vi "location_plot.vi"() -> ()   [LabVIEW 2016]
uses:
  <vilib>/sound2/lvsound2.llb/Sound Output Task ID.ctl
panel:
  in  "task ID 4":T1 format="%.0x"
  out "task ID out":T1 format="%.0x"
  out "error out 4":errorcluster
  in  "error in (no error) 4":errorcluster
  out "output 12":dbl
  in  "timeout (sec) 3":dbl
  in  "error in (no error) 3":errorcluster
  out "error out 3":errorcluster
  out "task ID 3":T1 format="%.0x"
  in  "timeout (sec) 2":dbl
  in  "error in (no error) 2":errorcluster
  out "error out 2":errorcluster
  out "task ID 2":T1 format="%.0x"
  out "Ball 5":cluster{"Color":string, "y":dbl, "x":dbl}
  out "Ball 4":cluster{"Color":string, "y":dbl, "x":dbl}
  out "Ball 3":cluster{"Color":string, "x":dbl, "y":dbl}
  out "Ball 2":cluster{"Color":string, "x":dbl, "y":dbl}
  out "ballcnt":dbl
  out "Ball 1":cluster{"Color":string, "x":dbl, "y":dbl}
  out "by":dbl
  out "task ID":T1 format="%.0x"
  out "error out":errorcluster
  in  "error in (no error)":errorcluster
  in  "timeout (sec)":dbl
  out "bx":dbl
  out "Numeric 2":dbl
  out "Numeric":dbl
  out "bflag":dbl
  out "pathy":dbl
  out "pathx":dbl
  out "object":dbl
  in  "stop":bool
  in  "Display History":bool
  out "2D Picture":picture
  in  "Size":i16=3
  out "bearing":dbl
  out "velocity":dbl
  out "Y":dbl
  out "X":dbl=5.0
  in  "DAC 2":dbl
  in  "DAC 1":dbl
  in  "Send Button":bool
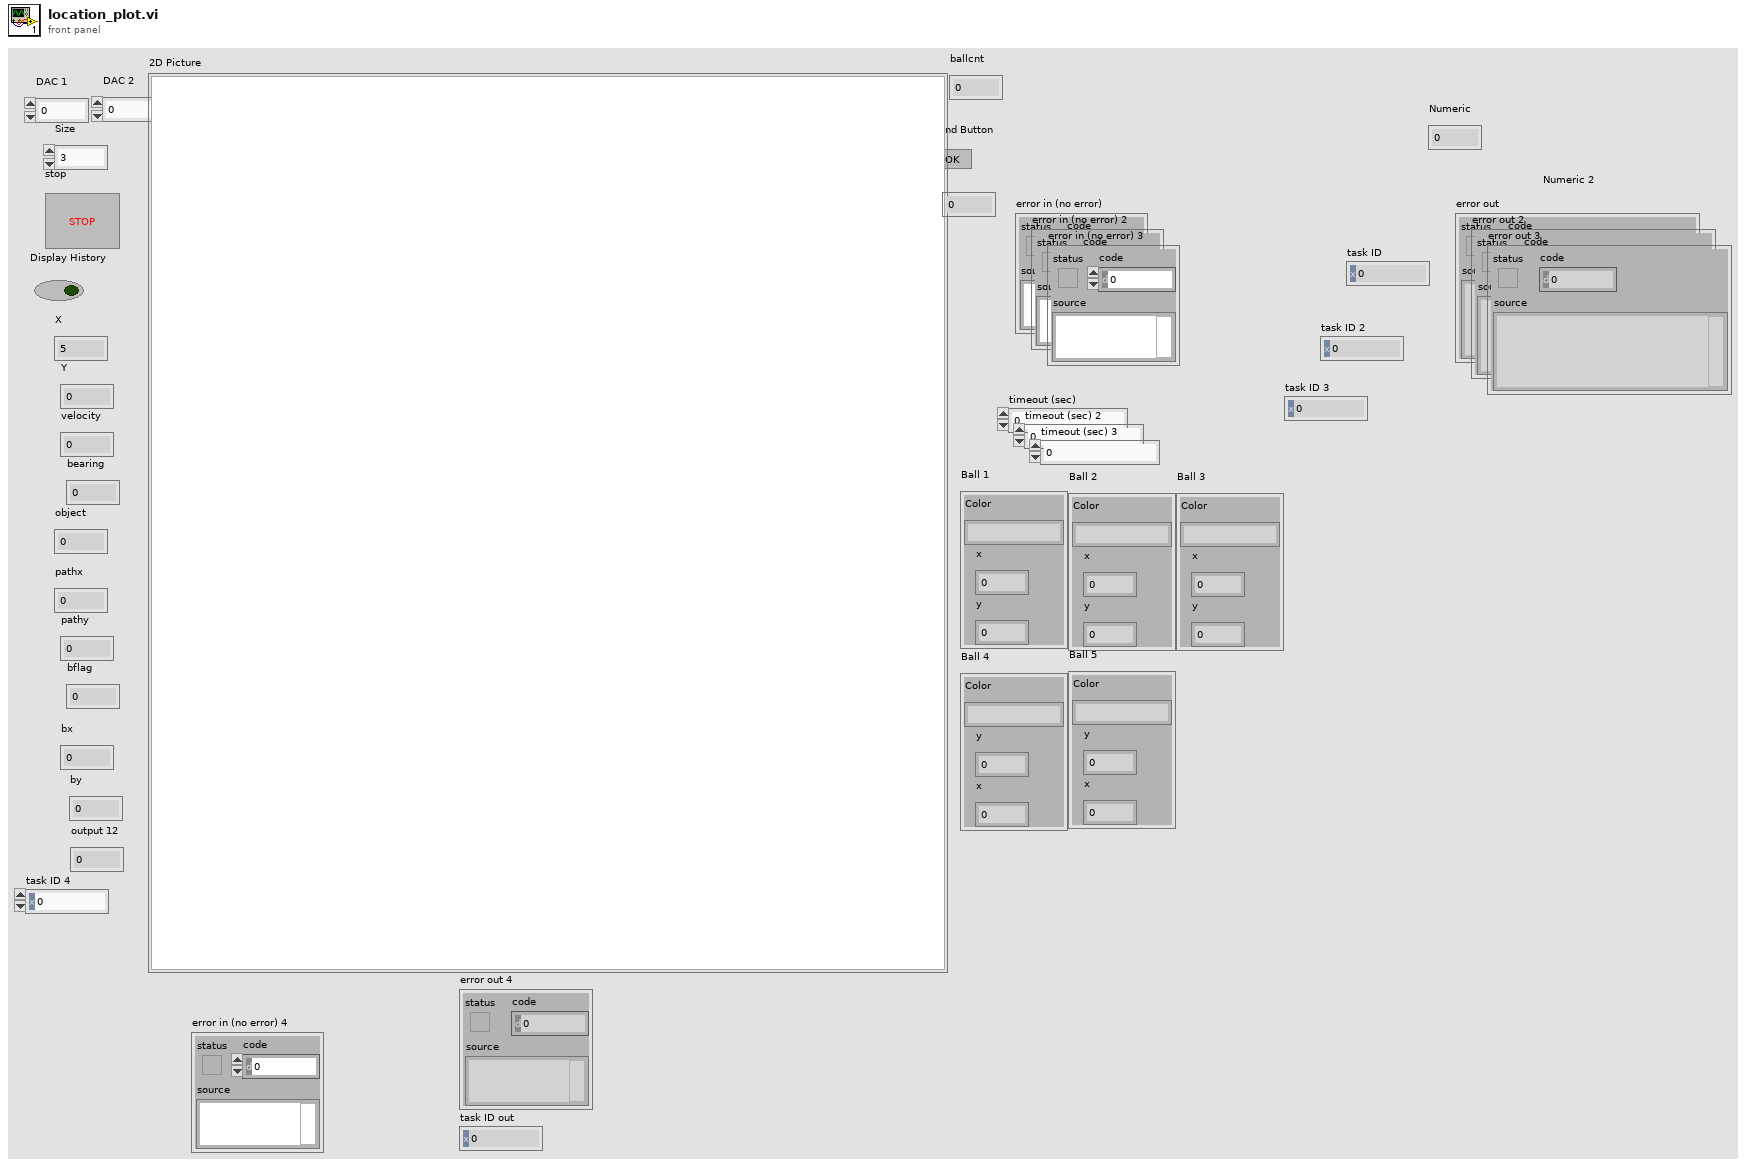
[diagram p1: front panel]
types:
  T1 = typedef "Sound Output Task ID.ctl" = u32
  T2 = cluster{"Width":u16, "Style":enum32{"Solid", "Dash", "Dot", "DashDot", "DashDotDot"}}
  T3 = enum16{"Standard", "Buffered", "CRLF", "Immediate"}
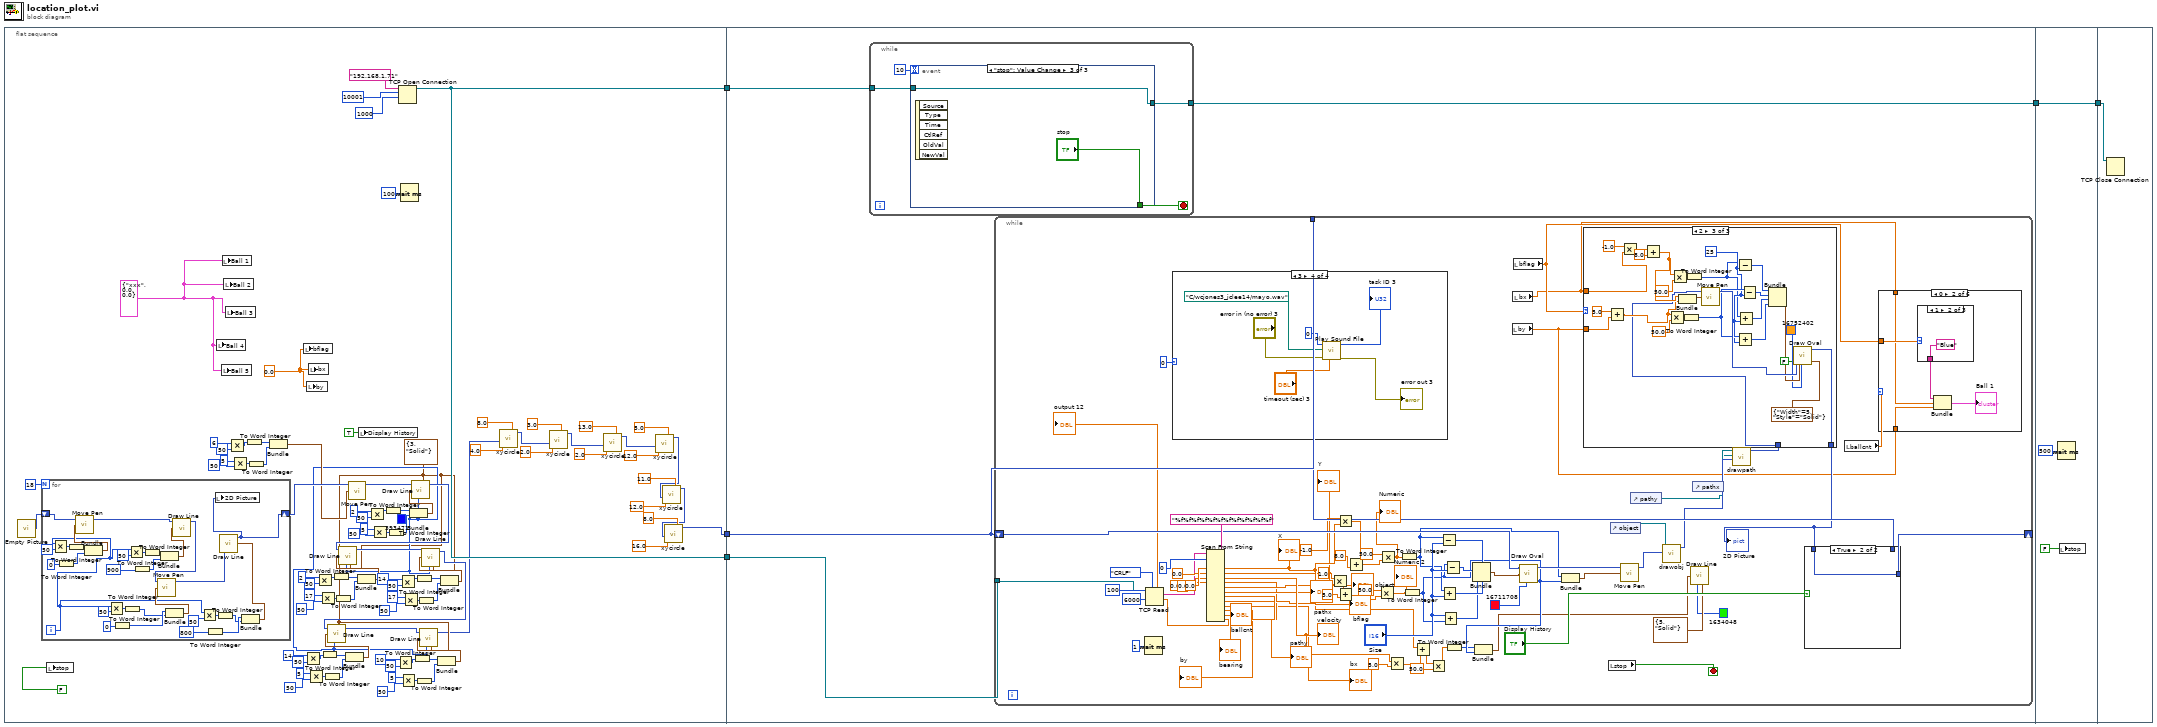
[diagram p0: block diagram]
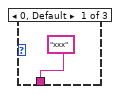
[diagram p3: hidden frame]
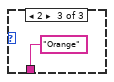
[diagram p4: hidden frame]
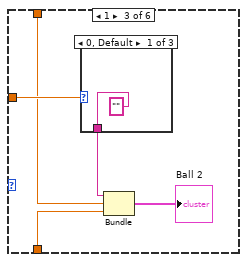
[diagram p5: hidden frame]
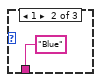
[diagram p6: hidden frame]
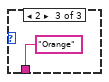
[diagram p7: hidden frame]
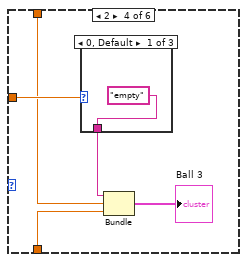
[diagram p8: hidden frame]
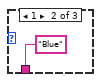
[diagram p9: hidden frame]
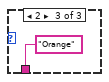
[diagram p10: hidden frame]
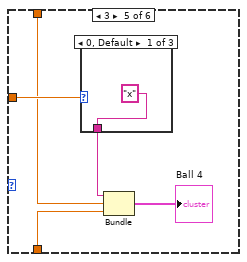
[diagram p11: hidden frame]
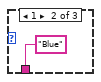
[diagram p12: hidden frame]
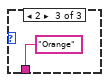
[diagram p13: hidden frame]
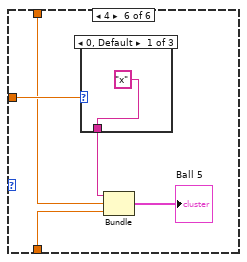
[diagram p14: hidden frame]
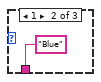
[diagram p15: hidden frame]
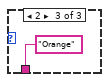
[diagram p16: hidden frame]
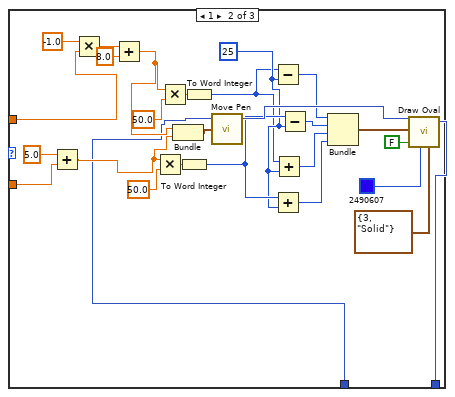
[diagram p18: hidden frame]
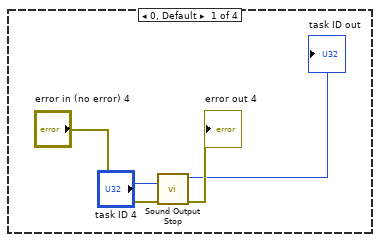
[diagram p19: hidden frame]
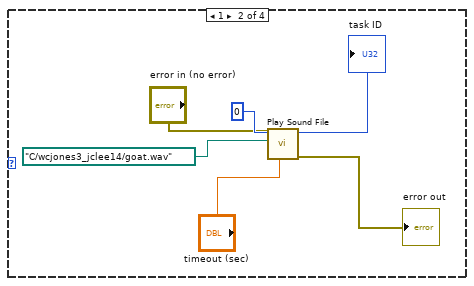
[diagram p20: hidden frame]
diagram:
  n1 = flat-sequence {
    tunnel: [w93] -> w5
    tunnel: [w93] -> w4
    tunnel: [w8] -> w1
    tunnel: w5 -> [w131]
    tunnel: w4 -> [w130]
    tunnel: [w129] -> w3
    tunnel: w1 -> [w128]
    tunnel: w3 -> [w344]
    tunnel: [w344] -> w2
    tunnel: w2 -> [w346]
    frame #0 {
      w6 = cluster{"Color":string, "x":dbl, "y":dbl} {"Color"="xxx", "x"=0.0, "y"=0.0} ("Ball 1")
      w7 = 0.0
      w27 = T2 {"Width"=3, "Style"=enum."Solid"} ("pen")
      w28 = u32 393471 ("color(black)")
      n2 = call "Empty Picture"() -> ("empty picture"=w89:picture)
      n3 = for {
        N: 18 -> [_]
        shift-right: [w100] -> w88
        shift-left: w89 -> [w99]
        i -> [w98]
        n4 = Multiply(x=w98, y=50) -> (x*y=w126:i32)
        n5 = To Word Integer(number=0) -> (16bit integer=w124:i16)
        n6 = To Word Integer(number=w126) -> (16bit integer=w123:i16)
        n7 = Bundle(w123, w124) -> (w122:cluster{i16, i16})  [unwired: 1 in]
        n8 = call <vilib>:"Move Pen.vi"("new position"=w122, "picture"=w99) -> ("new picture"=w115:picture)  [unwired: 3 in]
        n9 = Multiply(x=w98, y=50) -> (x*y=w108:i32)
        n10 = To Word Integer(number=0) -> (16bit integer=w106:i16)
        n11 = To Word Integer(number=w108) -> (16bit integer=w105:i16)
        n12 = Multiply(x=w98, y=50) -> (x*y=w118:i32)
        n13 = To Word Integer(number=900) -> (16bit integer=w120:i16)
        n14 = To Word Integer(number=w118) -> (16bit integer=w121:i16)
        n15 = Bundle(w121, w120) -> (w116:cluster{i16, i16})  [unwired: 1 in]
        n16 = Bundle(w106, w105) -> (w110:cluster{i16, i16})  [unwired: 1 in]
        n17 = call <vilib>:"Draw Line.vi"("picture"=w115, "end point"=w116) -> ("new picture"=w102:picture)  [unwired: 7 in]
        n18 = call <vilib>:"Move Pen.vi"("new position"=w110, "picture"=w102) -> ("new picture"=w101:picture)  [unwired: 3 in]
        n19 = Multiply(x=w98, y=50) -> (x*y=w112:i32)
        n20 = To Word Integer(number=800) -> (16bit integer=w104:i16)
        n21 = To Word Integer(number=w112) -> (16bit integer=w103:i16)
        n22 = Bundle(w104, w103) -> (w114:cluster{i16, i16})  [unwired: 1 in]
        n23 = call <vilib>:"Draw Line.vi"("picture"=w101, "end point"=w114) -> ("new picture"=w100:picture)  [unwired: 7 in]
        n24 = local write "2D Picture"(w100) -> ()
      }
      n25 = local write "stop"(FALSE ("stop")) -> ()
      n26 = local write "Ball 4"(w6) -> ()
      n27 = local write "Ball 5"(w6) -> ()
      n28 = local write "Ball 1"(w6) -> ()
      n29 = local write "Ball 2"(w6) -> ()
      n30 = local write "Ball 3"(w6) -> ()
      n31 = Multiply(x=6, y=50) -> (x*y=w80:i32)
      n32 = Multiply(x=5, y=50) -> (x*y=w85:i32)
      n33 = To Word Integer(number=w80) -> (16bit integer=w86:i16)
      n34 = To Word Integer(number=w85) -> (16bit integer=w87:i16)
      n35 = Bundle(w86, w87) -> (w79:cluster{i16, i16})  [unwired: 1 in]
      n36 = local write "bflag"(w7) -> ()
      n37 = Multiply(x=14, y=50) -> (x*y=w45:i32)
      n38 = local write "by"(w7) -> ()
      n39 = Multiply(x=5, y=50) -> (x*y=w49:i32)
      n40 = local write "bx"(w7) -> ()
      n41 = Multiply(x=2, y=50) -> (x*y=w63:i32)
      n42 = Multiply(x=17, y=50) -> (x*y=w67:i32)
      n43 = To Word Integer(number=w45) -> (16bit integer=w44:i16)
      n44 = To Word Integer(number=w49) -> (16bit integer=w50:i16)
      n45 = To Word Integer(number=w63) -> (16bit integer=w62:i16)
      n46 = To Word Integer(number=w67) -> (16bit integer=w68:i16)
      n47 = Bundle(w44, w50) -> (w43:cluster{i16, i16})  [unwired: 1 in]
      n48 = call <vilib>:"Move Pen.vi"("new position"=w79, "picture"=w88) -> ("new picture"=w78:picture)  [unwired: 3 in]
      n49 = Bundle(w62, w68) -> (w61:cluster{i16, i16})  [unwired: 1 in]
      n50 = local write "Display History"(TRUE ("Display History")) -> ()
      n51 = Multiply(x=2, y=50) -> (x*y=w77:i32)
      n52 = Multiply(x=5, y=50) -> (x*y=w72:i32)
      n53 = To Word Integer(number=w77) -> (16bit integer=w71:i16)
      n54 = To Word Integer(number=w72) -> (16bit integer=w70:i16)
      n55 = Multiply(x=10, y=50) -> (x*y=w35:i32)
      n56 = TCP Open Connection(address="192.168.1.71", remote port or service name=u16 10001, timeout ms (60000)=1000) -> (connection ID=w93:refnum<k5>)  [unwired: 2 in, 1 out]
      n57 = Multiply(x=14, y=50) -> (x*y=w57:i32)
      n58 = Multiply(x=5, y=50) -> (x*y=w31:i32)
      n59 = Wait (ms)(milliseconds to wait=u32 100) -> ()  [unwired: 1 out]
      n60 = Multiply(x=17, y=50) -> (x*y=w53:i32)
      n61 = Bundle(w71, w70) -> (w69:cluster{i16, i16})  [unwired: 1 in]
      n62 = call <vilib>:"Draw Line.vi"("picture"=w78, "end point"=w69, "color(black)"=w28, "pen"=w27) -> ("new picture"=w60:picture)  [unwired: 5 in]
      n63 = call <vilib>:"Draw Line.vi"("picture"=w60, "end point"=w61, "color(black)"=w28, "pen"=w27) -> ("new picture"=w51:picture)  [unwired: 5 in]
      n64 = To Word Integer(number=w35) -> (16bit integer=w36:i16)
      n65 = To Word Integer(number=w57) -> (16bit integer=w58:i16)
      n66 = To Word Integer(number=w31) -> (16bit integer=w30:i16)
      n67 = To Word Integer(number=w53) -> (16bit integer=w52:i16)
      n68 = Bundle(w36, w30) -> (w37:cluster{i16, i16})  [unwired: 1 in]
      n69 = Bundle(w58, w52) -> (w59:cluster{i16, i16})  [unwired: 1 in]
      n70 = call <vilib>:"Draw Line.vi"("picture"=w51, "end point"=w59, "color(black)"=w28, "pen"=w27) -> ("new picture"=w42:picture)  [unwired: 5 in]
      n71 = call <vilib>:"Draw Line.vi"("picture"=w42, "end point"=w43, "color(black)"=w28, "pen"=w27) -> ("new picture"=w29:picture)  [unwired: 5 in]
      n72 = call <vilib>:"Draw Line.vi"("picture"=w29, "end point"=w37, "color(black)"=w28, "pen"=w27) -> ("new picture"=w16:picture)  [unwired: 5 in]
      n73 = call "xycircle.vi"("new picture in"=w16, "y"=4.0, "x"=8.0) -> ("new picture out"=w15:picture)  [unwired: 8 in]
      n74 = call "xycircle.vi"("new picture in"=w15, "y"=2.0, "x"=3.0) -> ("new picture out"=w14:picture)  [unwired: 8 in]
      n75 = call "xycircle.vi"("new picture in"=w14, "y"=2.0, "x"=13.0) -> ("new picture out"=w13:picture)  [unwired: 8 in]
      n76 = call "xycircle.vi"("new picture in"=w13, "y"=12.0, "x"=5.0) -> ("new picture out"=w12:picture)  [unwired: 8 in]
      n77 = call "xycircle.vi"("new picture in"=w12, "y"=12.0, "x"=11.0) -> ("new picture out"=w9:picture)  [unwired: 8 in]
      n78 = call "xycircle.vi"("new picture in"=w9, "y"=16.0, "x"=8.0) -> ("new picture out"=w8:picture)  [unwired: 8 in]
    }
    frame #1 {
      n79 = while {
        tunnel: w131 -> [w326]
        tunnel: [w324] -> w129
        stop <- w327 stop-if-true
        n80 = event shown="[2] \"stop\": Value Change" {
          selector: _ -> [_ _ _]
          dyn-events: _ -> [_ _ _]
          timeout: 10 -> [_ _ _]
          tunnel: [FALSE FALSE "stop"] -> w327
          tunnel: w326 -> [w328 w332 w341]
          tunnel: [w328 w331 w341] -> w324
          event Timeout {
            n81 = event-data() -> ()  [unwired: 1 in, 3 out]
          }
          event "Send Button": Value Change {
            n82 = event-data() -> ()  [unwired: 1 in, 6 out]
            n83 = Format Into String(format string="%f %f", "DAC 1", "DAC 2") -> (resulting string=w337:string)  [unwired: 2 in, 1 out]
            n84 = Concatenate Strings("\\FD" ("string"), w337, "\\FF" ("string")) -> (w334:string)
            n85 = TCP Write(connection ID=w332, data in=w334, 9:100 ("timeout ms (25000)")) -> (connection ID out=w331:refnum<k5>)  [unwired: 1 in, 2 out]
          }
          event "stop": Value Change {
            n86 = event-data() -> ()  [unwired: 1 in, 6 out]
          }
        }
      }
      n87 = while {
        tunnel: w130 -> [w201]
        shift-right: [w183] -> _
        shift-left: w128 -> [w181]
        tunnel: w128 -> [w182]
        stop <- w184 stop-if-true
        n88 = Wait (ms)(milliseconds to wait=u32 1) -> ()  [unwired: 1 out]
        n89 = TCP Read(connection ID=w201, bytes to read=100, 7:T3."CRLF" ("mode (standard)"), 9:6000 ("timeout ms (25000)")) -> (data out=w193:string)  [unwired: 1 in, 2 out]
        n90 = case shown="3" 0 {
          frame 0, Default {
            n91 = call <vilib>:"Sound Output Stop.vi"("error in (no error)"="error in (no error) 4", "task ID"="task ID 4") -> ("error out"=→"error out 4":errorcluster, "task ID out"=→"task ID out":T1)  [unwired: 8 in]
          }
          frame 1 {
            n92 = call <vilib>:"Play Sound File.vi"("timeout (sec)"="timeout (sec)", "error in (no error)"="error in (no error)", "path"=path "C:/wcjones3_jclee14/goat.wav", "device ID"=u32 0) -> ("error out"=→"error out":errorcluster, "task ID"=→"task ID":T1)  [unwired: 6 in]
          }
          frame 2 {
            n93 = call <vilib>:"Play Sound File.vi"("timeout (sec)"="timeout (sec) 2", "error in (no error)"="error in (no error) 2", "path"=path "C:/wcjones3_jclee14/sendit.wav", "device ID"=u32 0) -> ("error out"=→"error out 2":errorcluster, "task ID"=→"task ID 2":T1)  [unwired: 6 in]
          }
          frame 3 {
            n94 = call <vilib>:"Play Sound File.vi"("timeout (sec)"="timeout (sec) 3", "error in (no error)"="error in (no error) 3", "path"=path "C:/wcjones3_jclee14/mayo.wav", "device ID"=u32 0) -> ("error out"=→"error out 3":errorcluster, "task ID"=→"task ID 3":T1)  [unwired: 6 in]
          }
        }
        n95 = Scan From String(format string="%f%f%f%f%f%f%f%f%f%f%f%f", input string=w193, initial scan location=u32 0, default 1=0.0 ("default value 1"), default 2=0.0 ("default value 2"), default 3=0.0 ("default value 3"), default 4=0.0 ("default value 4")) -> (output 1=w153:dbl, output 2=w150:dbl, output 3=w177:dbl, output 4=→"bearing":dbl, output 5=→"object":dbl, output 6=→"pathx":dbl, output 7=→"pathy":dbl, output 8=→"bflag":dbl, output 9=→"bx":dbl, output 10=→"by":dbl, output 11=→"ballcnt":dbl, output 12=→"output 12":dbl)  [unwired: 9 in, 3 out]
        "X" <- w153
        "Y" <- w150
        "velocity" <- w177
        n96 = Multiply(x=1.0, y=w150) -> (x*y=w151:dbl)
        n97 = Multiply(x=-1.0, y=w153) -> (x*y=w154:dbl)
        n98 = Add(x=w151, y=5.0) -> (x+y=w158:dbl)
        n99 = Add(x=w154, y=8.0) -> (x+y=w159:dbl)
        n100 = Multiply(x=50.0, y=w158) -> (x*y=w157:dbl)
        "Numeric 2" <- w157
        n101 = Multiply(x=50.0, y=w159) -> (x*y=w156:dbl)
        "Numeric" <- w156
        n102 = Multiply(x=w177, y=5.0) -> (x*y=w178:dbl)
        n103 = To Word Integer(number=w156) -> (16bit integer=w171:i16)
        n104 = To Word Integer(number=w157) -> (16bit integer=w170:i16)
        n105 = Add(x=w153, y=w178) -> (x+y=w166:dbl)
        n106 = Multiply(x=w166, y=50.0) -> (x*y=w167:dbl)
        n107 = Subtract(x=w171, y="Size") -> (x-y=w189:i16)
        n108 = Add(x=w171, y="Size") -> (x+y=w187:i16)
        n109 = Add(x="Size", y=w170) -> (x+y=w186:i16)
        n110 = Subtract(x=w170, y="Size") -> (x-y=w188:i16)
        n111 = To Word Integer(number=w167) -> (16bit integer=w169:i16)
        n112 = Bundle(w189, w188, w187, w186) -> (w180:cluster{i16, i16, i16, i16})  [unwired: 1 in]
        n113 = Bundle(w169, w170) -> (w168:cluster{i16, i16})  [unwired: 1 in]
        n114 = local read "by"() -> (w136:dbl)
        n115 = local read "bx"() -> (w137:dbl)
        n116 = local read "bflag"() -> (w138:dbl)
        n117 = call <vilib>:"Draw Oval.vi"("picture"=w181, "rect"=w180, "color(black)"=u32 16711708) -> ("new picture"=w175:picture)  [unwired: 6 in]
        n118 = Bundle(w171, w170) -> (w174:cluster{i16, i16})  [unwired: 1 in]
        n119 = local read "stop"() -> (w184:bool)
        n120 = control-ref of="object"() -> (w147:refnum<vi>)
        n121 = call <vilib>:"Move Pen.vi"("new position"=w174, "picture"=w175) -> ("new picture"=w148:picture)  [unwired: 3 in]
        n122 = control-ref of="pathy"() -> (w144:refnum<vi>)
        n123 = call "drawobj.vi"("new picture in"=w148, "Digital in"=w147) -> ("new picture out"=w146:picture)  [unwired: 9 in]
        n124 = call <vilib>:"Draw Line.vi"("end point"=w168, "color(black)"=u32 1634048, "pen"=T2 {"Width"=5, "Style"=enum."Solid"}) -> ()  [unwired: 6 in, 1 out]
        n125 = control-ref of="pathx"() -> (w145:refnum<vi>)
        n126 = call "drawpath.vi"("new picture in"=w146, "reference in"=w144, "Digital in"=w145) -> ("new picture"=w140:picture)  [unwired: 8 in]
        n127 = case shown="2" w138 {
          tunnel: w137 -> [_ w250 w275]
          tunnel: w136 -> [_ w249 w274]
          tunnel: w140 -> [w245 w248 w277]
          tunnel: [w245 w247 w273] -> w139
          frame 0, Default {
          }
          frame 1 {
            w264 = i16 25 ("Waypoint \nSize")
            n128 = Add(x=5.0, y=w249) -> (x+y=w252:dbl)
            n129 = Multiply(x=-1.0, y=w250) -> (x*y=w256:dbl)
            n130 = Add(x=w256, y=8.0) -> (x+y=w253:dbl)
            n131 = Multiply(x=w252, y=50.0) -> (x*y=w265:dbl)
            n132 = Multiply(x=w253, y=50.0) -> (x*y=w262:dbl)
            n133 = Bundle(w253, w252) -> (w270:cluster{dbl, dbl})  [unwired: 1 in]
            n134 = To Word Integer(number=w265) -> (16bit integer=w267:i16)
            n135 = To Word Integer(number=w262) -> (16bit integer=w263:i16)
            n136 = call <vilib>:"Move Pen.vi"("new position"=w270, "picture"=w248) -> ("new picture"=w271:picture)  [unwired: 3 in]
            n137 = Subtract(x=w263, y=w264) -> (x-y=w257:i16)
            n138 = Add(x=w267, y=w264) -> (x+y=w260:i16)
            n139 = Add(x=w263, y=w264) -> (x+y=w259:i16)
            n140 = Subtract(x=w267, y=w264) -> (x-y=w258:i16)
            n141 = Bundle(w257, w258, w259, w260) -> (w269:cluster{i16, i16, i16, i16})  [unwired: 1 in]
            n142 = call <vilib>:"Draw Oval.vi"("picture"=w271, "rect"=w269, "fill?(F)"=FALSE, "color(black)"=u32 2490607, "pen"=T2 {"Width"=3, "Style"=enum."Solid"}) -> ("new picture"=w247:picture)  [unwired: 4 in]
          }
          frame 2 {
            w291 = i16 25 ("Waypoint \nSize")
            n143 = Add(x=5.0, y=w274) -> (x+y=w279:dbl)
            n144 = Multiply(x=-1.0, y=w275) -> (x*y=w283:dbl)
            n145 = Add(x=w283, y=8.0) -> (x+y=w280:dbl)
            n146 = Multiply(x=w279, y=50.0) -> (x*y=w292:dbl)
            n147 = Multiply(x=w280, y=50.0) -> (x*y=w289:dbl)
            n148 = Bundle(w280, w279) -> (w297:cluster{dbl, dbl})  [unwired: 1 in]
            n149 = To Word Integer(number=w292) -> (16bit integer=w294:i16)
            n150 = To Word Integer(number=w289) -> (16bit integer=w290:i16)
            n151 = call <vilib>:"Move Pen.vi"("new position"=w297, "picture"=w277) -> ("new picture"=w298:picture)  [unwired: 3 in]
            n152 = Subtract(x=w290, y=w291) -> (x-y=w284:i16)
            n153 = Add(x=w294, y=w291) -> (x+y=w287:i16)
            n154 = Add(x=w290, y=w291) -> (x+y=w286:i16)
            n155 = Subtract(x=w294, y=w291) -> (x-y=w285:i16)
            n156 = Bundle(w284, w285, w286, w287) -> (w296:cluster{i16, i16, i16, i16})  [unwired: 1 in]
            n157 = call <vilib>:"Draw Oval.vi"("picture"=w298, "rect"=w296, "fill?(F)"=FALSE, "color(black)"=u32 16752402, "pen"=T2 {"Width"=5, "Style"=enum."Solid"}) -> ("new picture"=w273:picture)  [unwired: 4 in]
          }
        }
        "2D Picture" <- w139
        n158 = case shown="True" "Display History" {
          tunnel: [w322 w323] -> w183
          tunnel: w182 -> [w322 _]
          tunnel: w139 -> [_ w323]
          frame False {
          }
          frame True {
          }
        }
        n159 = local read "ballcnt"() -> (w134:dbl)
        n160 = case shown="0" w134 {
          tunnel: w138 -> [_ w208 w216 w224 w232 w240]
          tunnel: w137 -> [_ w207 w215 w223 w231 w239]
          tunnel: w136 -> [_ w206 w214 w222 w230 w238]
          frame -1, Default {
          }
          frame 0 {
            n161 = case shown="1" w208 {
              tunnel: ["xxx" "Blue" "Orange"] -> w209
              frame 0, Default {
              }
              frame 1 {
              }
              frame 2 {
              }
            }
            n162 = Bundle(w209, "bx"=w207, "by"=w206) -> (→"Ball 1":cluster{string, "bx":dbl, "by":dbl})  [unwired: 1 in]
          }
          frame 1 {
            n163 = case shown="0, Default" w216 {
              tunnel: ["" "Blue" "Orange"] -> w217
              frame 0, Default {
              }
              frame 1 {
              }
              frame 2 {
              }
            }
            n164 = Bundle(w217, "bx"=w215, "by"=w214) -> (→"Ball 2":cluster{string, "bx":dbl, "by":dbl})  [unwired: 1 in]
          }
          frame 2 {
            n165 = case shown="0, Default" w224 {
              tunnel: ["empty" "Blue" "Orange"] -> w225
              frame 0, Default {
              }
              frame 1 {
              }
              frame 2 {
              }
            }
            n166 = Bundle(w225, "bx"=w223, "by"=w222) -> (→"Ball 3":cluster{string, "bx":dbl, "by":dbl})  [unwired: 1 in]
          }
          frame 3 {
            n167 = case shown="0, Default" w232 {
              tunnel: ["x" "Blue" "Orange"] -> w233
              frame 0, Default {
              }
              frame 1 {
              }
              frame 2 {
              }
            }
            n168 = Bundle(w233, "bx"=w231, "by"=w230) -> (→"Ball 4":cluster{string, "bx":dbl, "by":dbl})  [unwired: 1 in]
          }
          frame 4 {
            n169 = case shown="0, Default" w240 {
              tunnel: ["x" "Blue" "Orange"] -> w241
              frame 0, Default {
              }
              frame 1 {
              }
              frame 2 {
              }
            }
            n170 = Bundle(w241, "bx"=w239, "by"=w238) -> (→"Ball 5":cluster{string, "bx":dbl, "by":dbl})  [unwired: 1 in]
          }
        }
      }
    }
    frame #2 {
      (unwired) FALSE ("stop")
      n171 = Wait (ms)(milliseconds to wait=u32 500) -> ()  [unwired: 1 out]
      n172 = local write "stop"(FALSE ("stop")) -> ()
    }
    frame #3 {
      n173 = TCP Close Connection(connection ID=w346) -> ()  [unwired: 2 in, 2 out]
    }
  }
